vi "编辑设定参数.vi"() -> ()   [LabVIEW 2018]
panel:
  in  "退出":bool
  in  "确定写入":bool
  out "Repeat_number":string="Repeat_number"
  out "Y_displacement":string="Y_displacement"
  out "X_displacement":string="X_displacement"
  out "X_Lowerr_value":string="Y_Lowerr_value"
  out "Y_Upper_value":string="Y_Upper_value"
  out "X_Lowerr_value":string="X Lowerr value"
  out "X_Upper_value":string="X_Upper_value"
  out "Deceleration_time":string="Deceleration time"
  out "Acceleration_time":string="Acceleration_time"
  out "Delay_Time":string="Delay_Time"
  in  "设定参数":string[][](array[string])
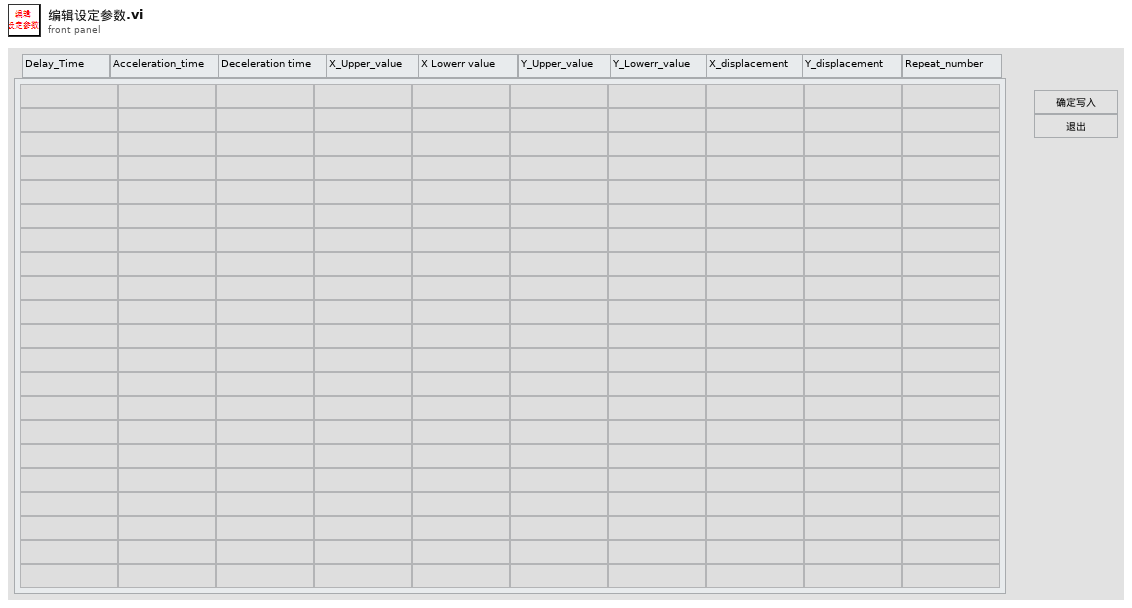
[diagram p1: front panel]
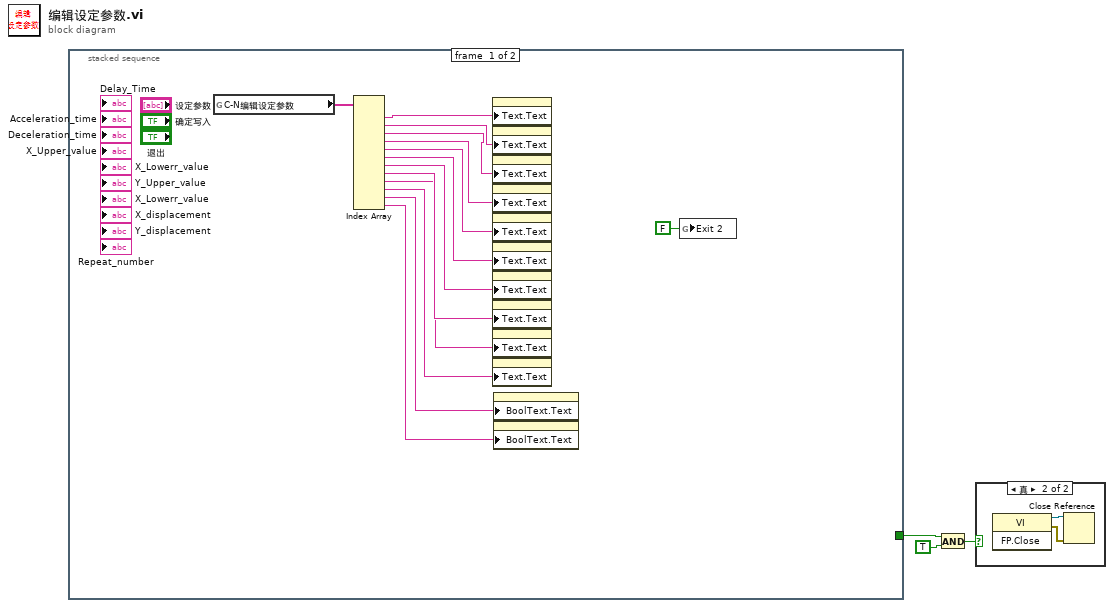
[diagram p0: block diagram]
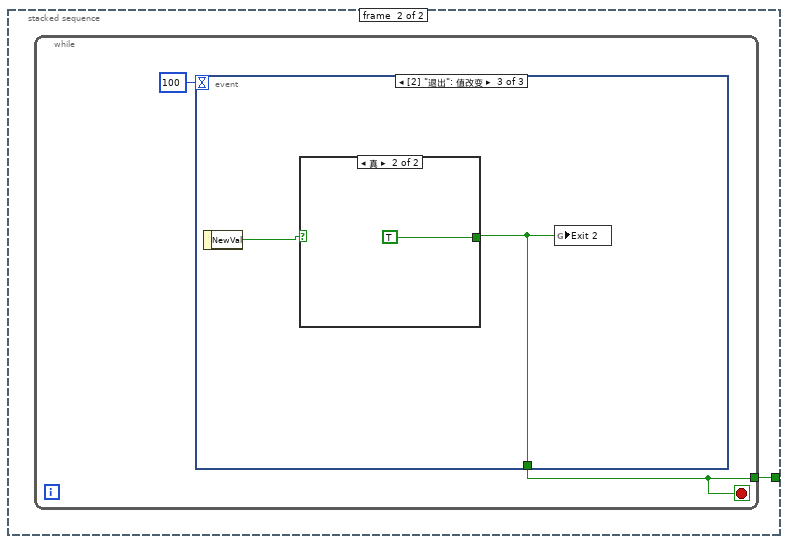
[diagram p2: hidden frame]
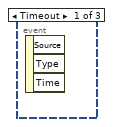
[diagram p3: hidden frame]
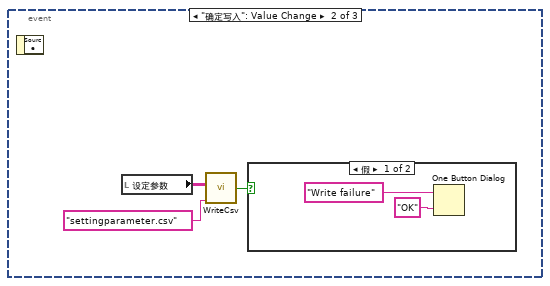
[diagram p4: hidden frame]
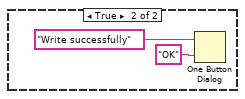
[diagram p5: hidden frame]
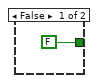
[diagram p6: hidden frame]
diagram:
  n1 = stacked-sequence {
    tunnel: [_ w18] -> w1
    frame #0 {
      n2 = global read "全局 1.vi" "C-N编辑设定参数"() -> (w17:string[])
      n3 = Index Array(array=w17) -> (element #1=w16:string, element #2=w15:string, element #3=w14:string, element #4=w13:string, element #5=w12:string, element #6=w11:string, element #7=w10:string, element #8=w9:string, element #9=w8:string, element #10=w7:string, element #11=w6:string, element #12=w5:string)  [unwired: 12 in]
      n4 = property on="Delay_Time" class="Str"("Text.Text"=w16) -> ()  [unwired: 2 in, 2 out]
      n5 = property on="Acceleration_time" class="Str"("Text.Text"=w15) -> ()  [unwired: 2 in, 2 out]
      n6 = property on="Deceleration_time" class="Str"("Text.Text"=w14) -> ()  [unwired: 2 in, 2 out]
      n7 = property on="X_Upper_value" class="Str"("Text.Text"=w13) -> ()  [unwired: 2 in, 2 out]
      n8 = property on="X_Lowerr_value" class="Str"("Text.Text"=w12) -> ()  [unwired: 2 in, 2 out]
      n9 = property on="Y_Upper_value" class="Str"("Text.Text"=w11) -> ()  [unwired: 2 in, 2 out]
      n10 = property on="X_Lowerr_value" class="Str"("Text.Text"=w10) -> ()  [unwired: 2 in, 2 out]
      n11 = property on="X_displacement" class="Str"("Text.Text"=w9) -> ()  [unwired: 2 in, 2 out]
      n12 = property on="Y_displacement" class="Str"("Text.Text"=w8) -> ()  [unwired: 2 in, 2 out]
      n13 = property on="Repeat_number" class="Str"("Text.Text"=w7) -> ()  [unwired: 2 in, 2 out]
      n14 = property on="确定写入" class="Bool"("BoolText.Text"=w6) -> ()  [unwired: 2 in, 2 out]
      n15 = property on="退出" class="Bool"("BoolText.Text"=w5) -> ()  [unwired: 2 in, 2 out]
      n16 = global write "全局 1.vi" "Exit 2"(FALSE ("Exit 2")) -> ()
    }
    frame #1 {
      n17 = while {
        tunnel: [w19] -> w18
        stop <- w19 stop-if-true
        n18 = event shown="[2] \"退出\": 值改变" {
          selector: _ -> [_ _ _]
          dyn-events: _ -> [_ _ _]
          timeout: 100 -> [_ _ _]
          tunnel: [_ _ w28] -> w19
          event Timeout {
            n19 = event-data() -> ()  [unwired: 1 in, 3 out]
          }
          event "确定写入": Value Change {
            n20 = event-data() -> ()  [unwired: 1 in, 1 out]
            n21 = local read "设定参数"() -> (w22:string[][])
            n22 = call "WriteCsv.vi"("相对路径"="settingparameter.csv", "2D data"=w22) -> ("布尔"=w21:bool)  [unwired: 2 in]
            n23 = case shown="假" w21 {
              frame False {
                n24 = One Button Dialog(message="Write failure" ("消息"), button name ("OK")="OK" ("按钮名称（“确定”）")) -> ()  [unwired: 1 out]
              }
              frame True {
                n25 = One Button Dialog(message="Write successfully" ("消息"), button name ("OK")="OK" ("按钮名称（“确定”）")) -> ()  [unwired: 1 out]
              }
            }
          }
          event "退出": Value Change {
            n26 = event-data() -> ("NewVal"=w29:bool)  [unwired: 1 in]
            n27 = case shown="真" w29 {
              tunnel: [FALSE TRUE] -> w28
              frame False {
              }
              frame True {
              }
            }
            n28 = global write "全局 1.vi" "Exit 2"(w28) -> ()
          }
        }
      }
    }
  }
  n29 = And(x=w1, y=TRUE) -> (x .and. y?=w2:bool)
  n30 = case shown="真" w2 {
    frame False {
    }
    frame True {
      n31 = invoke class="VI" method="FP.Close"() -> (reference out=w33:refnum<vi>, error out=w32:errorcluster)  [unwired: 3 in, 1 out]
      n32 = Close Reference(reference=w33, error in (no error)=w32) -> ()  [unwired: 1 out]
    }
  }
